vi "Enqueue_Queue_Single.vi"(6 "Prioty":bool, 8 "error in (no error)":errorcluster, 9 "Data":variant, 10 "Command":string, 11 "queue In":refnum<queue>) -> (0 "error out":errorcluster, 3 "queue Out":refnum<queue>)   [LabVIEW 2014, in "Queue_Library.lvlib"]
uses:
  Queue_Library.lvlib
  TypeDef.ctl
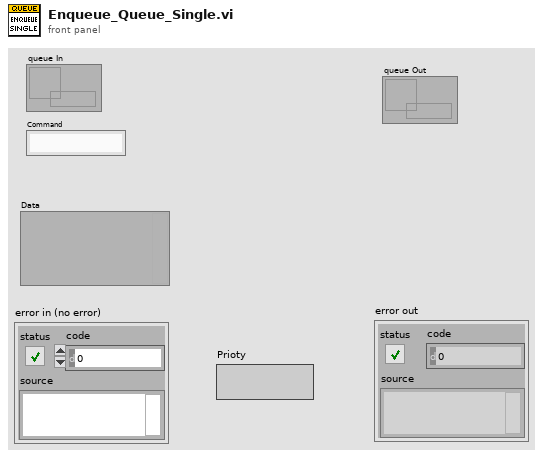
[diagram p1: front panel]
types:
  T1 = typedef "Queue_Library.lvlib/TypeDef.ctl" = cluster{"Command":string, "Data":variant}
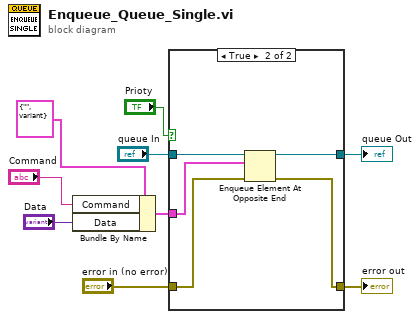
[diagram p0: block diagram]
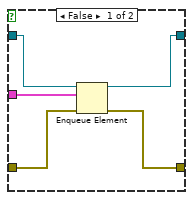
[diagram p2: hidden frame]
diagram:
  n1 = Bundle By Name(cluster=T1 {"Command"="", "Data"=variant} ("Message"), "Command"="Command", "Data"="Data") -> (w4:T1)
  n2 = case shown="True" "Prioty" {
    tunnel: [w14 w18] -> w7
    tunnel: "error in (no error)" -> [w13 w19]
    tunnel: w4 -> [w12 w17]
    tunnel: "queue In" -> [w10 w16]
    tunnel: [w11 w15] -> w1
    frame False {
      n3 = Enqueue Element(queue=w10, element=w12, error in (no error)=w13) -> (queue out=w11:refnum<queue>, error out=w14:errorcluster)  [unwired: 1 in, 1 out]
    }
    frame True {
      n4 = Enqueue Element At Opposite End(queue=w16, element=w17, error in (no error)=w19) -> (queue out=w15:refnum<queue>, error out=w18:errorcluster)  [unwired: 1 in, 1 out]
    }
  }
  "error out" <- w7
  "queue Out" <- w1
